vi "IMU RECORDER_AU_2024_v4.vi"() -> ()   [LabVIEW 2021]
uses:
  IMU data typedef.ctl
  <vilib>/Utility/sysdir.llb/System Directory Type.ctl
panel:
  out "TDMS REC!":bool
  in  "Run":bool caption="Run deluje le ob zagonu programa,\nda se zagotovi, da najprej izbereš port.\nÈe program ustaviš s tipko stop, moraš \nza ponoven zagon program še enkrat odpret."
  out "RT REC ID":i32
  in  "Tab Control 2":T1(tab)
  out "LostPackets":cluster{"f":dbl, "f":dbl}(graph)={"f"=1.0, "f"=0.0}
  out "LPR":cluster{dbl, dbl}(graph)={100.0, 0.0}
  out "BATT":cluster{"Ubat 1":dbl, "Ubat 2":dbl}(graph)
  out "Ubat 1":dbl
  out "IMU Temp 1":dbl=25.0
  out "DATA 1":string
  out "Stop IMU 1":bool
  in  "IMU port 1":u16=2000
  in  "T=last value, F=zero 1L":bool=TRUE
  out "Timeout 1":bool=TRUE
  out "IMU1 - 6D":refnum<k16>
  out "IMU DATA 1":T2
  out "IMU DATA 2":T2={"ACCEL-X"=1.0213841634214662, "ACCEL-Y"=0.0, "ACCEL-Z"=0.0, "GYRO - X"=0.0, "GYRO - Y"=0.0, "GYRO - Z"=0.0, "MAG-Z"=0.0, "MAG-Y"=0.0, "MAG-X"=0.0, "TEMP"=0.0, "BATT"=0.0, "RAW DATA"="|A| T:   394897 Ax:   2093 Ay: END\u0000", "TIMESTAMP"=394897.0}
  in  "IMU port 2":u16=1234
  out "DATA 2":string
  out "IMU2 - 6D":refnum<k16>
  in  "T=last value, F=zero 1L 2":bool=TRUE caption="T=last value, F=zero 1L"
  out "Timeout 2":bool
  out "Stop IMU 2":bool
  out "LiPo MIN":dbl=3.4
  out "LiPo NOM":dbl=3.7
  out "F1":bool
  out "A1":bool=TRUE
  in  "stop 1":bool
  in  "stop 2":bool
  out "IMU Temp 2":dbl=25.0
  out "Ubat 2":dbl
  out "F2":bool
  out "A2":bool=TRUE
  out "GYRO 2":T3(graph)={"AVG(X,N)"=-1.87176, "AVG(X,N)"=2.10976, "AVG(X,N)"=1.55397}
  out "ACC 2":T3(graph)={"AVG(X,N)"=0.9979845636557063, "AVG(X,N)"=-0.031232, "AVG(X,N)"=0.0110239}
  out "GYRO 1":T3(graph)={"AVG(X,N)"=-1.87176, "AVG(X,N)"=1.48327, "AVG(X,N)"=2.96304}
  in  "IMU CHART":bool=TRUE
  in  "CAL IMU2":bool
  out "BIAS 1":T4={"ACCEL-X"=0.0236778, "ACCEL-Y"=0.0366586, "ACCEL-Z"=-0.00184464, "GYRO - X"=1.87176, "GYRO - Y"=-1.48327, "GYRO - Z"=-2.96304, "TIMESTAMP"=0.0}
  out "BIAS 2":T4={"ACCEL-X"=0.0248636, "ACCEL-Y"=0.031232, "ACCEL-Z"=-0.0110239, "GYRO - X"=1.87176, "GYRO - Y"=-2.10976, "GYRO - Z"=-1.55397, "TIMESTAMP"=0.0}
  out "ACC 1":T3(graph)={"AVG(X,N)"=-0.0236778, "AVG(X,N)"=-0.0366586, "AVG(X,N)"=0.00184464}
  in  "CAL IMU1":bool
  in  "N_BIAS_IMU":i32=100
  out "date/time string":string="2024_03_08"
  out "ShrambaLabview":path=path "C:/Users/toneu/TDMS"
  out "Lokacija shranjevanja":path=path "C:/Users/toneu/TDMS/2024_03_08"
  in  "sample time":u32=5
  out "LV TimeStamp":i32=3689096
  out "sample ID":i32=2027
  out "ovd":bool
  out "system directory":path=path "C:/Users/toneu"
  out "Dt":cluster{dbl, dbl, dbl}(graph)={6.0, 0.0, 4.0}
  out "AbsAcc":cluster{"magnitude":dbl, "magnitude":dbl}(graph)={"magnitude"=0.04367944440500131, "magnitude"=0.9965830780399628}
  out "Seconds":i32=10 format="%.2f"
  out "REC FileName":string="IMU-06-06-18-13-48.tdms"
  out "TMP File Name":string="D-03-08-14-46-22.tdms"
  in  "RECORD":bool
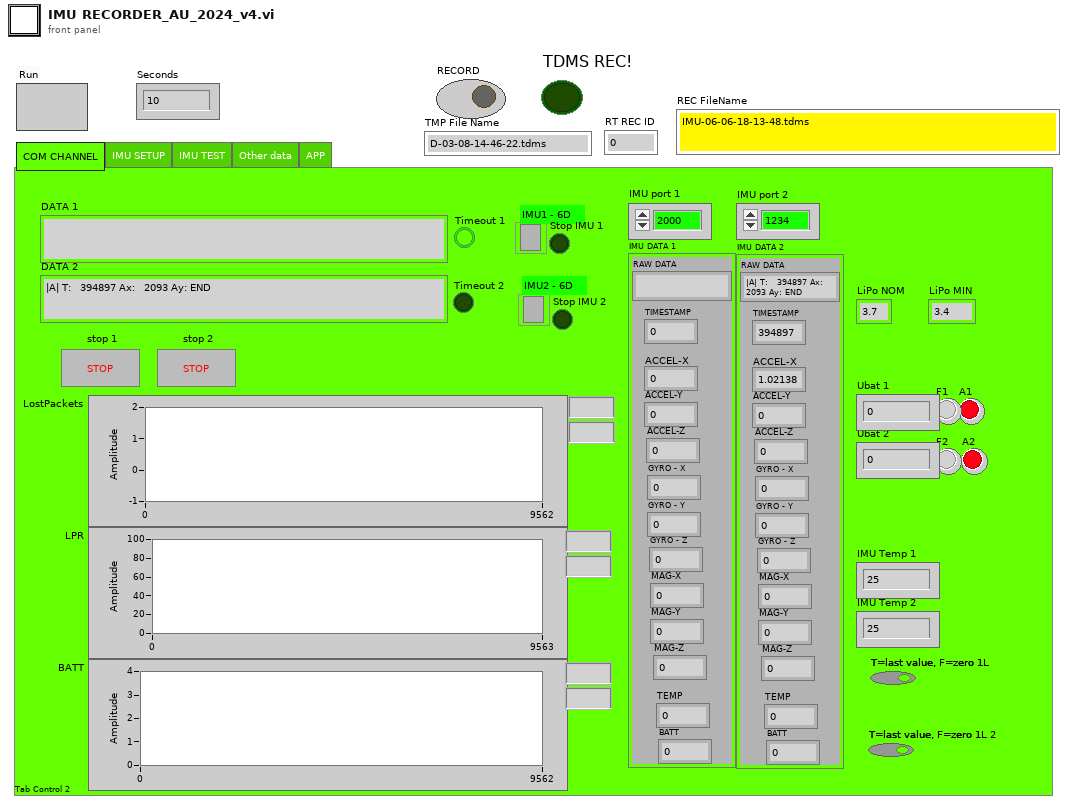
[diagram p1: front panel]
types:
  T1 = enum32{"COM CHANNEL", "IMU SETUP", "IMU TEST", "Other data", "APP"}
  T2 = typedef "IMU data typedef.ctl" = cluster{"ACCEL-X":dbl, "ACCEL-Y":dbl, "ACCEL-Z":dbl, "GYRO - X":dbl, "GYRO - Y":dbl, "GYRO - Z":dbl, "MAG-Z":dbl, "MAG-Y":dbl, "MAG-X":dbl, "TEMP":dbl, "BATT":dbl, "RAW DATA":string, "TIMESTAMP":dbl}
  T3 = cluster{"AVG(X,N)":dbl, "AVG(X,N)":dbl, "AVG(X,N)":dbl}
  T4 = cluster{"ACCEL-X":dbl, "ACCEL-Y":dbl, "ACCEL-Z":dbl, "GYRO - X":dbl, "GYRO - Y":dbl, "GYRO - Z":dbl, "TIMESTAMP":dbl}
  T5 = typedef "System Directory Type.ctl" = i32
  T6 = cluster{"ACCEL-X":dbl, "ACCEL-Y":dbl, "ACCEL-Z":dbl}
  T7 = cluster{"GYRO - X":dbl, "GYRO - Y":dbl, "GYRO - Z":dbl}
  T8 = cluster{"AVG(X,N)":dbl, "AVG(X,N)":dbl, dbl, "AVG(X,N)":dbl, "AVG(X,N)":dbl, "AVG(X,N)":dbl, "y":dbl}
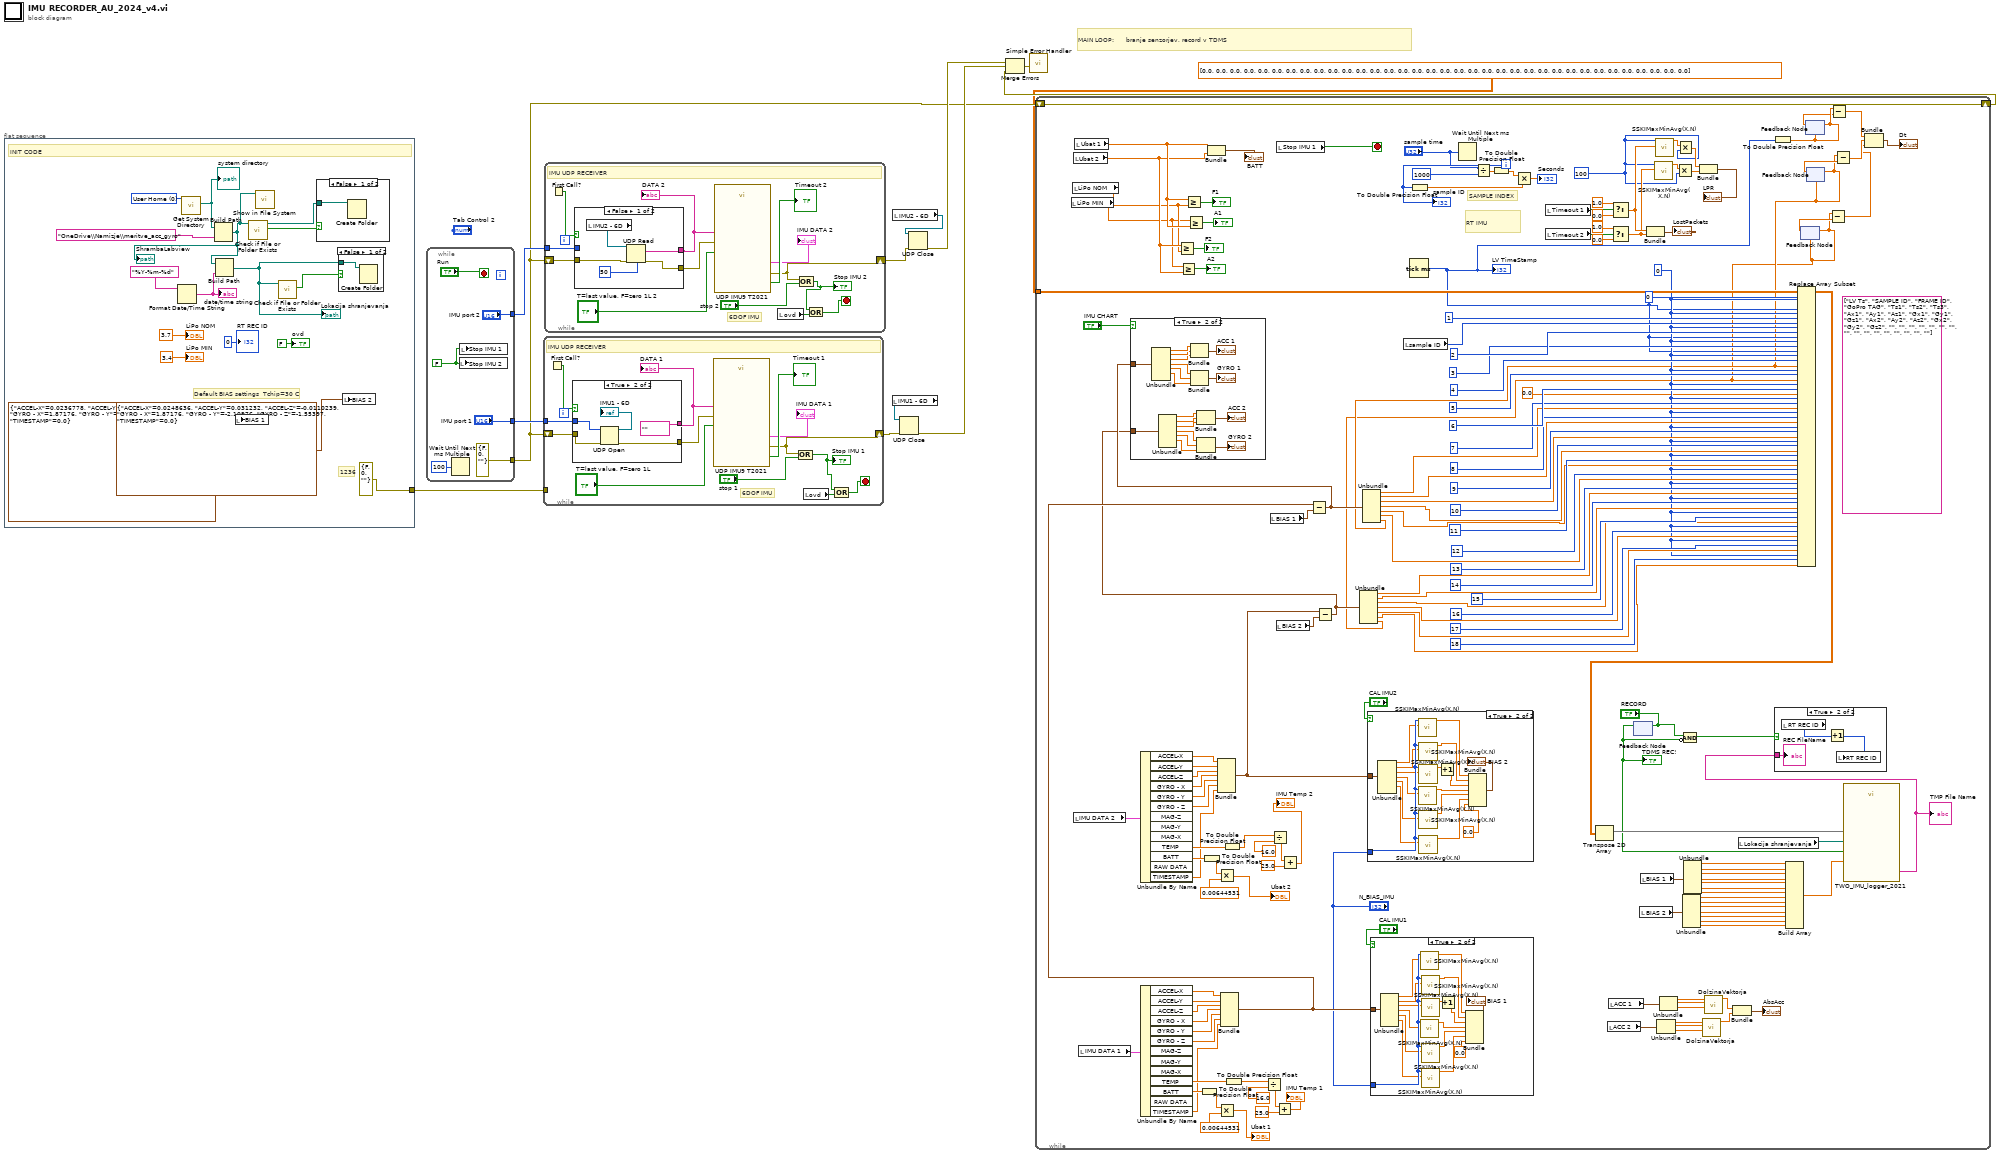
[diagram p0: block diagram]
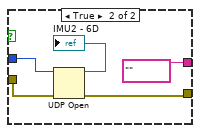
[diagram p2: hidden frame]
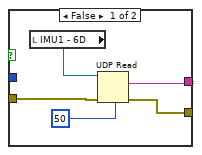
[diagram p9: hidden frame]
diagram:
  # "MAIN LOOP:      branje senzorjev, record v TDMS"
  n1 = flat-sequence {
    tunnel: [errorcluster {"status"=FALSE, "code"=0, "source"=""} ("error constant")] -> w8
    frame #0 {
      w14 = T5 0 items=["User Home"=0, "User Desktop"=1, "User Documents"=2, "User Application Data"=3, "User Preferences"=4, "User Temporary"=5, "Public Documents"=6, "Public Application Data"=7, "Public Preferences"=8, "Public Cache"=13, "System Core Libraries"=9, "System Installed Libraries"=10, "Application Files"=11, "Boot Volume Root"=12] ("system directory type")
      # "1236"
      # "Default BIAS settings  Tchip=30 C"
      # "1235"
      # "INIT CODE"
      n2 = Format Date/Time String(time format string (%c)="%Y-%m-%d") -> (date/time string=w21:string)  [unwired: 2 in]
      "date/time string" <- w21
      n3 = call <vilib>:"Get System Directory.vi"("system directory type"=w14) -> ("system directory"=w19:path)  [unwired: 10 in]
      "system directory" <- w19
      n4 = Build Path(base path=w19, name or relative path="OneDrive\\Namizje\\meritve_acc_gyro") -> (appended path=w24:path)
      "ShrambaLabview" <- w24
      n5 = Build Path(base path=w24, name or relative path=w21) -> (appended path=w23:path)
      "Lokacija shranjevanja" <- w23
      n6 = local write "BIAS 1"(T4 {"ACCEL-X"=0.0236778, "ACCEL-Y"=0.0366586, "ACCEL-Z"=-0.00184464, "GYRO - X"=1.87176, "GYRO - Y"=-1.48327, "GYRO - Z"=-2.96304, "TIMESTAMP"=0.0} ("output cluster")) -> ()
      n7 = call <vilib>:"Check if File or Folder Exists.vi"("path"=w24) -> ("file or folder exists?"=w18:bool, "dup path"=w20:path)  [unwired: 8 in, 1 out]
      n8 = call <vilib>:"Show in File System.vi"("file or directory path"=w24) -> ()  [unwired: 10 in, 1 out]
      n9 = call <vilib>:"Check if File or Folder Exists.vi"("path"=w23) -> ("file or folder exists?"=w22:bool)  [unwired: 8 in, 2 out]
      n10 = case shown="False" w18 {
        tunnel: w20 -> [w32 _]
        frame False {
          n11 = Create Folder(path (use dialog)=w32) -> ()  [unwired: 2 in, 3 out]
        }
        frame True {
        }
      }
      n12 = case shown="False" w22 {
        tunnel: w23 -> [w31 _]
        frame False {
          n13 = Create Folder(path (use dialog)=w31) -> ()  [unwired: 2 in, 3 out]
        }
        frame True {
        }
      }
      n14 = local write "BIAS 2"(T4 {"ACCEL-X"=0.0248636, "ACCEL-Y"=0.031232, "ACCEL-Z"=-0.0110239, "GYRO - X"=1.87176, "GYRO - Y"=-2.10976, "GYRO - Z"=-1.55397, "TIMESTAMP"=0.0} ("output cluster")) -> ()
      "LiPo NOM" <- 3.7 ("LiPo MIN")
      "LiPo MIN" <- 3.4 ("LiPo MIN")
      "RT REC ID" <- 0 ("Trig sample ID")
      "ovd" <- FALSE ("ovd")
    }
  }
  n15 = while {
    tunnel: [errorcluster {"status"=FALSE, "code"=0, "source"=""} ("error constant")] -> w2
    tunnel: ["IMU port 1"] -> w10
    tunnel: ["IMU port 2"] -> w4
    stop <- "Run" stop-if-true
    w33 = FALSE ("Stopping...")
    n16 = Wait Until Next ms Multiple(millisecond multiple=u32 100) -> ()  [unwired: 1 out]
    n17 = local write "Stop IMU 2"(w33) -> ()
    n18 = local write "Stop IMU 1"(w33) -> ()
  }
  n19 = while {
    tunnel: w10 -> [w49]
    shift-right: [w46] -> w11
    shift-left: w2 -> [w48]
    tunnel: w8 -> [_]
    stop <- w40 stop-if-true
    # "6DOF IMU"
    # "IMU UDP RECEIVER"
    n20 = First Call?() -> (First Call?: T/F=w50:bool)
    n21 = case shown="True" w50 {
      tunnel: w49 -> [_ w61]
      tunnel: w48 -> [w54 w59]
      tunnel: [w53 w58] -> w44
      tunnel: [w52 "" ("data out")] -> w45
      frame False {
        n22 = local read "IMU1 - 6D"() -> (w56:refnum<k16>)
        n23 = UDP Read(connection ID=w56, timeout ms (25000)=50, 8:w54) -> (data out=w52:string, error out=w53:errorcluster)  [unwired: 4 out]
      }
      frame True {
        n24 = UDP Open(8:w59, 11:w61) -> (port=→"IMU1 - 6D":refnum<k16>, 0:w58:errorcluster)  [unwired: 3 in, 1 out]
      }
    }
    "DATA 1" <- w45
    n25 = call "UDP IMU9 T2021.vi"("T=last value, F=zero"="T=last value, F=zero 1L", "Error In"=w44, "data in"=w45) -> ("Error Out"=w46:errorcluster, "Data Out"=→"IMU DATA 1":T2, "Timeout"=→"Timeout 1":bool)  [unwired: 6 in]
    n26 = Compound Arithmetic op=OR(w46, "stop 1") -> (w39:bool)
    "Stop IMU 1" <- w39
    n27 = local read "ovd"() -> (w41:bool)
    n28 = Compound Arithmetic op=OR(w39, w41) -> (w40:bool)
  }
  n29 = while {
    tunnel: w4 -> [w72]
    shift-right: [w69] -> w6
    shift-left: w2 -> [w71]
    stop <- w64 stop-if-true
    # "6DOF IMU"
    # "IMU UDP RECEIVER"
    n30 = First Call?() -> (First Call?: T/F=w73:bool)
    n31 = case shown="False" w73 {
      tunnel: w72 -> [_ w84]
      tunnel: w71 -> [w77 w82]
      tunnel: [w76 w81] -> w67
      tunnel: [w75 "" ("data out")] -> w68
      frame False {
        n32 = local read "IMU2 - 6D"() -> (w79:refnum<k16>)
        n33 = UDP Read(connection ID=w79, timeout ms (25000)=50, 8:w77) -> (data out=w75:string, error out=w76:errorcluster)  [unwired: 4 out]
      }
      frame True {
        n34 = UDP Open(8:w82, 11:w84) -> (port=→"IMU2 - 6D":refnum<k16>, 0:w81:errorcluster)  [unwired: 3 in, 1 out]
      }
    }
    "DATA 2" <- w68
    n35 = call "UDP IMU9 T2021.vi"("T=last value, F=zero"="T=last value, F=zero 1L 2", "Error In"=w67, "data in"=w68) -> ("Error Out"=w69:errorcluster, "Data Out"=→"IMU DATA 2":T2, "Timeout"=→"Timeout 2":bool)  [unwired: 6 in]
    n36 = local read "ovd"() -> (w62:bool)
    n37 = Compound Arithmetic op=OR(w69, "stop 2") -> (w63:bool)
    "Stop IMU 2" <- w63
    n38 = Compound Arithmetic op=OR(w63, w62) -> (w64:bool)
  }
  n39 = local read "IMU1 - 6D"() -> (w12:refnum<k16>)
  n40 = local read "IMU2 - 6D"() -> (w3:refnum<k16>)
  n41 = UDP Close(connection ID=w12, 8:w11) -> (error out=w13:errorcluster)  [unwired: 1 out]
  n42 = UDP Close(connection ID=w3, 8:w6) -> (error out=w5:errorcluster)  [unwired: 1 out]
  n43 = while {
    tunnel: dbl[][] [[0.0, 0.0, 0.0, 0.0, 0.0, 0.0, 0.0, 0.0, 0.0, 0.0, 0.0, 0.0, 0.0, 0.0, 0.0, 0.0, 0.0, 0.0, 0.0, 0.0, 0.0, 0.0, 0.0, 0.0, 0.0, 0.0, 0.0, 0.0, 0.0, 0.0, 0.0, 0.0, 0.0, 0.0, 0.0]] ("LOG REC data") -> [w243]
    shift-right: [w226] -> w7
    shift-left: w2 -> [w226]
    i -> [w218]
    stop <- w225 stop-if-true
    (unwired) string[] ["LV Ts", "SAMPLE ID", "FRAME ID", "GoPro TAG", "Ts1", "Ts2", "Ts3", "Ax1", "Ay1", "Az1", "Gx1", "Gy1", "Gz1", "Ax2", "Ay2", "Az2", "Gx2", "Gy2", "Gz2", "", "", "", "", "", "", "", "", "", "", "", "", "", "", "", ""] ("channel name(s) in (Untitled)")
    w125 = 100 ("INT_ N")
    w121 = 0 ("disabled index (row)")
    # "SAMPLE INDEX"
    # "RT IMU"
    n44 = local read "LiPo MIN"() -> (w116:dbl)
    n45 = local read "LiPo NOM"() -> (w117:dbl)
    n46 = local read "Ubat 2"() -> (w118:dbl)
    n47 = local read "IMU DATA 2"() -> (w182:T2)
    n48 = local read "Ubat 1"() -> (w122:dbl)
    n49 = local read "IMU DATA 1"() -> (w195:T2)
    n50 = Unbundle By Name(w182) -> ("ACCEL-X"=w188:dbl, "ACCEL-Y"=w187:dbl, "ACCEL-Z"=w186:dbl, "GYRO - X"=w183:dbl, "GYRO - Y"=w184:dbl, "GYRO - Z"=w185:dbl, "TEMP"=w181:dbl, "BATT"=w180:dbl, "TIMESTAMP"=w172:dbl)  [unwired: 4 out]
    n51 = Unbundle By Name(w195) -> ("ACCEL-X"=w189:dbl, "ACCEL-Y"=w190:dbl, "ACCEL-Z"=w191:dbl, "GYRO - X"=w194:dbl, "GYRO - Y"=w193:dbl, "GYRO - Z"=w192:dbl, "TEMP"=w202:dbl, "BATT"=w203:dbl, "TIMESTAMP"=w173:dbl)  [unwired: 4 out]
    n52 = Greater Or Equal?(x=w118, y=w117) -> (x >= y?=→"F2":bool)
    n53 = Greater Or Equal?(x=w116, y=w118) -> (x >= y?=→"A2":bool)
    n54 = Greater Or Equal?(x=w122, y=w117) -> (x >= y?=→"F1":bool)
    n55 = Greater Or Equal?(x=w116, y=w122) -> (x >= y?=→"A1":bool)
    n56 = To Double Precision Float(number=w203) -> (double precision float=w220:dbl)
    n57 = To Double Precision Float(number=w180) -> (double precision float=w178:dbl)
    n58 = Bundle("Ubat 1"=w122, "Ubat 2"=w118) -> (→"BATT":cluster{"Ubat 1":dbl, "Ubat 2":dbl})  [unwired: 1 in]
    n59 = Bundle("ACCEL-X"=w188, "ACCEL-Y"=w187, "ACCEL-Z"=w186, "GYRO - X"=w183, "GYRO - Y"=w184, "GYRO - Z"=w185, "TIMESTAMP"=w172) -> (w111:T4)  [unwired: 1 in]
    n60 = Multiply(x=w178, y=0.00644531) -> (x*y=→"Ubat 2":dbl)
    n61 = Multiply(x=w220, y=0.00644531) -> (x*y=→"Ubat 1":dbl)
    n62 = Bundle("ACCEL-X"=w189, "ACCEL-Y"=w190, "ACCEL-Z"=w191, "GYRO - X"=w194, "GYRO - Y"=w193, "GYRO - Z"=w192, "TIMESTAMP"=w173) -> (w115:T4)  [unwired: 1 in]
    n63 = To Double Precision Float(number=w181) -> (double precision float=w136:dbl)
    n64 = To Double Precision Float(number=w202) -> (double precision float=w219:dbl)
    n65 = Divide(x=w219, y=16.0) -> (x/y=w223:dbl)
    n66 = local read "BIAS 1"() -> (w154:T4)
    n67 = Divide(x=w136, y=16.0) -> (x/y=w175:dbl)
    n68 = Add(x=w223, y=25.0) -> (x+y=→"IMU Temp 1":dbl)
    n69 = local read "BIAS 2"() -> (w153:T4)
    n70 = local read "Stop IMU 1"() -> (w225:bool)
    n71 = Add(x=w175, y=25.0) -> (x+y=→"IMU Temp 2":dbl)
    n72 = Subtract(x=w115, y=w154) -> (x-y=w108:T4)
    n73 = Subtract(x=w111, y=w153) -> (x-y=w107:T4)
    n74 = case shown="True" "IMU CHART" {
      tunnel: w108 -> [_ w291]
      tunnel: w107 -> [_ w284]
      frame False {
      }
      frame True {
        n75 = Unbundle(w291) -> ("ACCEL-X"=w297:dbl, "ACCEL-Y"=w296:dbl, "ACCEL-Z"=w295:dbl, "GYRO - X"=w294:dbl, "GYRO - Y"=w293:dbl, "GYRO - Z"=w292:dbl)  [unwired: 1 out]
        n76 = Unbundle(w284) -> ("ACCEL-X"=w285:dbl, "ACCEL-Y"=w286:dbl, "ACCEL-Z"=w287:dbl, "GYRO - X"=w288:dbl, "GYRO - Y"=w289:dbl, "GYRO - Z"=w290:dbl)  [unwired: 1 out]
        n77 = Bundle("ACCEL-X"=w297, "ACCEL-Y"=w296, "ACCEL-Z"=w295) -> (→"ACC 1":T6)  [unwired: 1 in]
        n78 = Bundle("GYRO - X"=w294, "GYRO - Y"=w293, "GYRO - Z"=w292) -> (→"GYRO 1":T7)  [unwired: 1 in]
        n79 = Bundle("ACCEL-X"=w285, "ACCEL-Y"=w286, "ACCEL-Z"=w287) -> (→"ACC 2":T6)  [unwired: 1 in]
        n80 = Bundle("GYRO - X"=w288, "GYRO - Y"=w289, "GYRO - Z"=w290) -> (→"GYRO 2":T7)  [unwired: 1 in]
      }
    }
    n81 = Unbundle(w107) -> ("ACCEL-X"=w165:dbl, "ACCEL-Y"=w163:dbl, "ACCEL-Z"=w161:dbl, "GYRO - X"=w159:dbl, "GYRO - Y"=w157:dbl, "GYRO - Z"=w155:dbl, "TIMESTAMP"=w85:dbl)
    n82 = Unbundle(w108) -> ("ACCEL-X"=w171:dbl, "ACCEL-Y"=w170:dbl, "ACCEL-Z"=w169:dbl, "GYRO - X"=w168:dbl, "GYRO - Y"=w167:dbl, "GYRO - Z"=w166:dbl, "TIMESTAMP"=w91:dbl)
    n83 = case shown="True" "CAL IMU2" {
      tunnel: "N_BIAS_IMU" -> [_ w261]
      tunnel: w111 -> [_ w254]
      frame False {
      }
      frame True {
        n84 = Unbundle(w254) -> ("ACCEL-X"=w260:dbl, "ACCEL-Y"=w259:dbl, "ACCEL-Z"=w258:dbl, "GYRO - X"=w257:dbl, "GYRO - Y"=w256:dbl, "GYRO - Z"=w255:dbl)  [unwired: 1 out]
        n85 = call "SSKIMaxMinAvg(X,N).vi"("X"=w260, "INT_ N"=w261) -> ("AVG(X,N)"=w253:dbl)  [unwired: 5 in, 4 out]
        n86 = call "SSKIMaxMinAvg(X,N).vi"("X"=w257, "INT_ N"=w261) -> ("AVG(X,N)"=w251:dbl)  [unwired: 5 in, 4 out]
        n87 = call "SSKIMaxMinAvg(X,N).vi"("X"=w259, "INT_ N"=w261) -> ("AVG(X,N)"=w252:dbl)  [unwired: 5 in, 4 out]
        n88 = call "SSKIMaxMinAvg(X,N).vi"("X"=w258, "INT_ N"=w261) -> ("AVG(X,N)"=w246:dbl)  [unwired: 5 in, 4 out]
        n89 = call "SSKIMaxMinAvg(X,N).vi"("X"=w256, "INT_ N"=w261) -> ("AVG(X,N)"=w250:dbl)  [unwired: 5 in, 4 out]
        n90 = call "SSKIMaxMinAvg(X,N).vi"("X"=w255, "INT_ N"=w261) -> ("AVG(X,N)"=w249:dbl)  [unwired: 5 in, 4 out]
        n91 = Increment(x=w246) -> (x+1=w245:dbl)
        n92 = Bundle("AVG(X,N)"=w253, "AVG(X,N)"=w252, w245, "AVG(X,N)"=w251, "AVG(X,N)"=w250, "AVG(X,N)"=w249, "y"=0.0) -> (→"BIAS 2":T8)  [unwired: 1 in]
      }
    }
    n93 = case shown="True" "CAL IMU1" {
      tunnel: "N_BIAS_IMU" -> [_ w278]
      tunnel: w115 -> [_ w271]
      frame False {
      }
      frame True {
        n94 = Unbundle(w271) -> ("ACCEL-X"=w277:dbl, "ACCEL-Y"=w276:dbl, "ACCEL-Z"=w275:dbl, "GYRO - X"=w274:dbl, "GYRO - Y"=w273:dbl, "GYRO - Z"=w272:dbl)  [unwired: 1 out]
        n95 = call "SSKIMaxMinAvg(X,N).vi"("X"=w277, "INT_ N"=w278) -> ("AVG(X,N)"=w270:dbl)  [unwired: 5 in, 4 out]
        n96 = call "SSKIMaxMinAvg(X,N).vi"("X"=w274, "INT_ N"=w278) -> ("AVG(X,N)"=w268:dbl)  [unwired: 5 in, 4 out]
        n97 = call "SSKIMaxMinAvg(X,N).vi"("X"=w276, "INT_ N"=w278) -> ("AVG(X,N)"=w269:dbl)  [unwired: 5 in, 4 out]
        n98 = call "SSKIMaxMinAvg(X,N).vi"("X"=w275, "INT_ N"=w278) -> ("AVG(X,N)"=w263:dbl)  [unwired: 5 in, 4 out]
        n99 = call "SSKIMaxMinAvg(X,N).vi"("X"=w273, "INT_ N"=w278) -> ("AVG(X,N)"=w267:dbl)  [unwired: 5 in, 4 out]
        n100 = call "SSKIMaxMinAvg(X,N).vi"("X"=w272, "INT_ N"=w278) -> ("AVG(X,N)"=w266:dbl)  [unwired: 5 in, 4 out]
        n101 = Increment(x=w263) -> (x+1=w262:dbl)
        n102 = Bundle("AVG(X,N)"=w270, "AVG(X,N)"=w269, w262, "AVG(X,N)"=w268, "AVG(X,N)"=w267, "AVG(X,N)"=w266, "y"=0.0) -> (→"BIAS 1":T8)  [unwired: 1 in]
      }
    }
    n103 = local read "sample ID"() -> (w201:i32)
    n104 = Tick Count (ms)() -> (millisecond timer value=w93:u32)
    "LV TimeStamp" <- w93
    n105 = To Double Precision Float(number=w218) -> (double precision float=w217:dbl)
    n106 = Wait Until Next ms Multiple(millisecond multiple="sample time") -> ()  [unwired: 1 out]
    n107 = Divide(x="sample time", y=i64 1000) -> (x/y=w216:dbl)
    n108 = To Double Precision Float(number=w216) -> (double precision float=w215:dbl)
    n109 = Multiply(x=w215, y=w217) -> (x*y=→"Seconds":dbl)
    n110 = local read "Timeout 1"() -> (w207:bool)
    n111 = local read "Timeout 2"() -> (w134:bool)
    n112 = local read "ACC 2"() -> (w99:T3)
    n113 = local read "ACC 1"() -> (w106:T3)
    n114 = Select(t=1.0, s=w207, f=0.0) -> (s? t:f=w130:dbl)
    n115 = Select(t=1.0, s=w134, f=0.0) -> (s? t:f=w129:dbl)
    n116 = feedback-in #1("RECORD") -> ()
    n117 = feedback #1() -> (w197:bool)  [unwired: 1 in]
    "TDMS REC!" <- w197
    n118 = local read "BIAS 2"() -> (w144:T4)
    n119 = local read "BIAS 1"() -> (w152:T4)
    n120 = Bundle("f"=w130, "f"=w129) -> (→"LostPackets":cluster{"f":dbl, "f":dbl})  [unwired: 1 in]
    n121 = call "SSKIMaxMinAvg(X,N).vi"("X"=w129, "INT_ N"=w125) -> ("AVG(X,N)"=w206:dbl)  [unwired: 5 in, 4 out]
    n122 = call "SSKIMaxMinAvg(X,N).vi"("X"=w130, "INT_ N"=w125) -> ("AVG(X,N)"=w128:dbl)  [unwired: 5 in, 4 out]
    n123 = Unbundle(w99) -> ("AVG(X,N)"=w100:dbl, "AVG(X,N)"=w101:dbl, "AVG(X,N)"=w102:dbl)
    n124 = Unbundle(w106) -> ("AVG(X,N)"=w105:dbl, "AVG(X,N)"=w104:dbl, "AVG(X,N)"=w103:dbl)
    n125 = Multiply(x=w206, y=w125) -> (x*y=w127:dbl)
    n126 = Multiply(x=w128, y=w125) -> (x*y=w126:dbl)
    n127 = Unbundle(w144) -> ("ACCEL-X"=w143:dbl, "ACCEL-Y"=w142:dbl, "ACCEL-Z"=w141:dbl, "GYRO - X"=w140:dbl, "GYRO - Y"=w139:dbl, "GYRO - Z"=w138:dbl, "TIMESTAMP"=w137:dbl)
    n128 = Compound Arithmetic op=AND("RECORD", invert w197) -> (w209:bool)
    n129 = Unbundle(w152) -> ("ACCEL-X"=w151:dbl, "ACCEL-Y"=w150:dbl, "ACCEL-Z"=w149:dbl, "GYRO - X"=w148:dbl, "GYRO - Y"=w147:dbl, "GYRO - Z"=w146:dbl, "TIMESTAMP"=w145:dbl)
    n130 = Bundle(w126, w127) -> (→"LPR":cluster{dbl, dbl})  [unwired: 1 in]
    n131 = call "DolzinaVektorja.vi"("z"=w102, "y"=w101, "x"=w100) -> ("magnitude"=w97:dbl)  [unwired: 8 in]
    n132 = call "DolzinaVektorja.vi"("z"=w103, "y"=w104, "x"=w105) -> ("magnitude"=w98:dbl)  [unwired: 8 in]
    n133 = Bundle("magnitude"=w98, "magnitude"=w97) -> (→"AbsAcc":cluster{"magnitude":dbl, "magnitude":dbl})  [unwired: 1 in]
    n134 = local read "Lokacija shranjevanja"() -> (w198:path)
    n135 = To Double Precision Float(number=w93) -> (double precision float=w95:dbl)
    n136 = Build Array(w151, w150, w149, w148, w147, w146, w145, w143, w142, w141, w140, w139, w138, w137) -> (w196:dbl[])
    n137 = Replace Array Subset(array=w243, new element #1=w93, index (row) #1=w121, index (col) #1=0 ("index"), new element #2=w201, index (row) #2=w121, index (col) #2=1 ("index"), new element #3=w93, index (row) #3=w121, index (col) #3=2 ("index"), new element #4=w93, index (row) #4=w121, index (col) #4=3 ("index"), new element #5=w91, index (row) #5=w121, index (col) #5=4 ("index"), new element #6=w85, index (row) #6=w121, index (col) #6=5 ("index"), new element #7=0.0 ("new element/subarray"), index (row) #7=w121, index (col) #7=6 ("index"), new element #8=w171, index (row) #8=w121, index (col) #8=7 ("index"), new element #9=w170, index (row) #9=w121, index (col) #9=8 ("index"), new element #10=w169, index (row) #10=w121, index (col) #10=9 ("index"), new element #11=w168, index (row) #11=w121, index (col) #11=10 ("index"), new element #12=w167, index (row) #12=w121, index (col) #12=11 ("index"), new element #13=w166, index (row) #13=w121, index (col) #13=12 ("index"), new element #14=w165, index (row) #14=w121, index (col) #14=13 ("index"), new element #15=w163, index (row) #15=w121, index (col) #15=14 ("index"), new element #16=w161, index (row) #16=w121, index (col) #16=15 ("index"), new element #17=w159, index (row) #17=w121, index (col) #17=16 ("index"), new element #18=w157, index (row) #18=w121, index (col) #18=17 ("index"), new element #19=w155, index (row) #19=w121, index (col) #19=18 ("index")) -> (w241:dbl[][])
    n138 = Transpose 2D Array(2D array=w241) -> (transposed array=w240:dbl[][])
    n139 = feedback #2(w85) -> (w87:dbl)
    n140 = feedback-in #2(w85) -> ()
    n141 = feedback #3(w95) -> (w94:dbl)
    n142 = feedback-in #3(w95) -> ()
    n143 = feedback #4(w91) -> (w92:dbl)
    n144 = feedback-in #4(w91) -> ()
    n145 = Subtract(x=w85, y=w87) -> (x-y=w86:dbl)
    n146 = Subtract(x=w95, y=w94) -> (x-y=w90:dbl)
    n147 = Subtract(x=w91, y=w92) -> (x-y=w89:dbl)
    n148 = call "TWO_IMU_logger_2021.vi"("PARAMETERS"=w196, "Folder"=w198, "LOG"=w197, "DATA"=w240) -> ("FileName"=w208:string)  [unwired: 7 in]
    "TMP File Name" <- w208
    n149 = case shown="True" w209 {
      tunnel: w208 -> [_ w281]
      frame False {
      }
      frame True {
        n150 = local read "RT REC ID"() -> (w280:i32)
        n151 = Increment(x=w280) -> (x+1=w279:i32)
        n152 = local write "RT REC ID"(w279) -> ()
        "REC FileName" <- w281
      }
    }
    n153 = Bundle(w90, w89, w86) -> (→"Dt":cluster{dbl, dbl, dbl})  [unwired: 1 in]
    "sample ID" <- w218
  }
  n154 = Merge Errors(w5, w13, w7) -> (w9:errorcluster)
  n155 = call <vilib>:"Simple Error Handler.vi"("error in (no error)"=w9) -> ()  [unwired: 1 in, 8 out]
